vi "Reset_VI_Connections.vi"(11 "expId":string) -> ()   [LabVIEW 2014]
doc: "Initializes to 0 the counter for the experiment VIs connections and disconnections"
uses:
  Configuration/Global_Configurations.vi
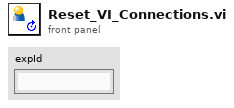
[diagram p1: front panel]
types:
  T1 = cluster{"Path":path, "Name":string, "Authors":string, "Keywords":string, "Description":string, "Cameras":cluster{"Base URL":string, "Path":string, "Name":string}[]}[]
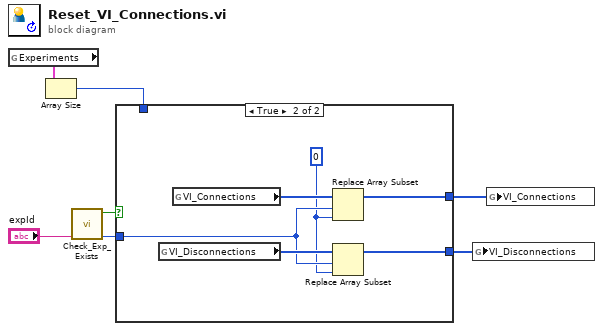
[diagram p0: block diagram]
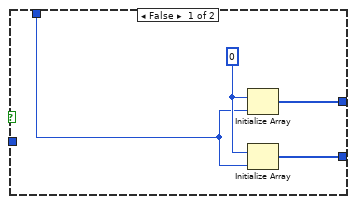
[diagram p2: hidden frame]
diagram:
  n1 = global read "Global_Configurations.vi" "Experiments"() -> (w2:T1)
  n2 = Array Size(array=w2) -> (size(s)=w1:i32)
  n3 = call "Check_Exp_Exists.vi"("expId"="expId") -> ("expIndex"=w3:i32, "exists"=w5:bool)  [unwired: 9 in]
  n4 = case shown="True" w5 {
    tunnel: [w11 w14] -> w7
    tunnel: [w10 w13] -> w6
    tunnel: w3 -> [_ w15]
    tunnel: w1 -> [w8 _]
    frame False {
      w9 = u8 0
      n5 = Initialize Array(w9, w8) -> (w11:u8[])
      n6 = Initialize Array(w9, w8) -> (w10:u8[])
    }
    frame True {
      w12 = u8 0 ("new element/subarray")
      n7 = global read "Global_Configurations.vi" "VI_Disconnections"() -> (w16:u8[])
      n8 = global read "Global_Configurations.vi" "VI_Connections"() -> (w17:u8[])
      n9 = Replace Array Subset(array=w17, new element=w12, index=w15) -> (w14:u8[])
      n10 = Replace Array Subset(array=w16, new element=w12, index=w15) -> (w13:u8[])
    }
  }
  n11 = global write "Global_Configurations.vi" "VI_Disconnections"(w6) -> ()
  n12 = global write "Global_Configurations.vi" "VI_Connections"(w7) -> ()
